vi "Read Config.vi"(8 "error in (no error)":errorcluster, 11 "HtmlReportPlugin in":refnum<class "HtmlReportPlugin.lvclass">) -> (0 "error out":errorcluster, 2 "Config":variant, 3 "HtmlReportPlugin out":refnum<class "HtmlReportPlugin.lvclass">)   [LabVIEW 2015, in "HtmlReportPlugin.lvclass"]
uses:
  HtmlReportPlugin.lvclass
  HtmlReportPlugin.lvclass/HtmlReportPlugin.ctl
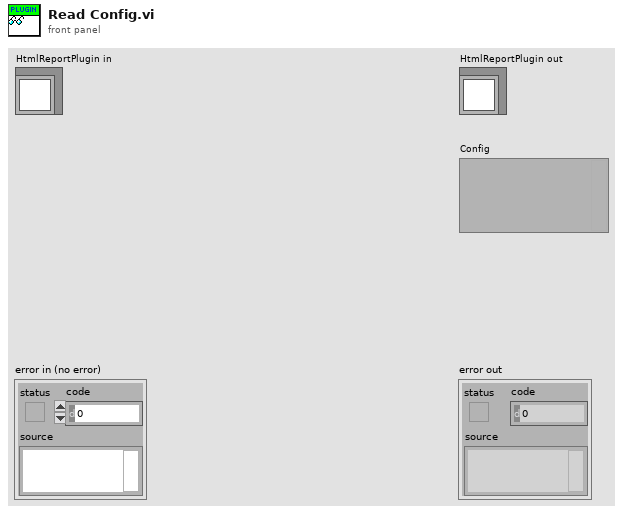
[diagram p1: front panel]
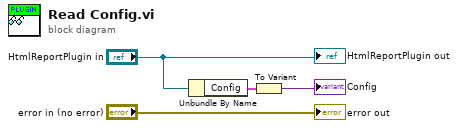
[diagram p0: block diagram]
diagram:
  n1 = Unbundle By Name("HtmlReportPlugin in") -> ("Config"=w4:cluster{"Enable":bool, "Report Folder":string})
  n2 = To Variant(anything=w4) -> (Variant=→"Config":variant)
  "error out" <- "error in (no error)"
  "HtmlReportPlugin out" <- "HtmlReportPlugin in"
